vi "graph drivable paths.vi"(2 "updated max path lengths":u16[](array[numeric]), 3 "possible wheel angles":i8[](array[numeric])=[0, 0, 0, 0, 0, 0, 0, 0, 0, 0, 0, 0, 0, 0, 0, 0]) -> (0 "XY Graph":T1(graph))   [LabVIEW 2010]
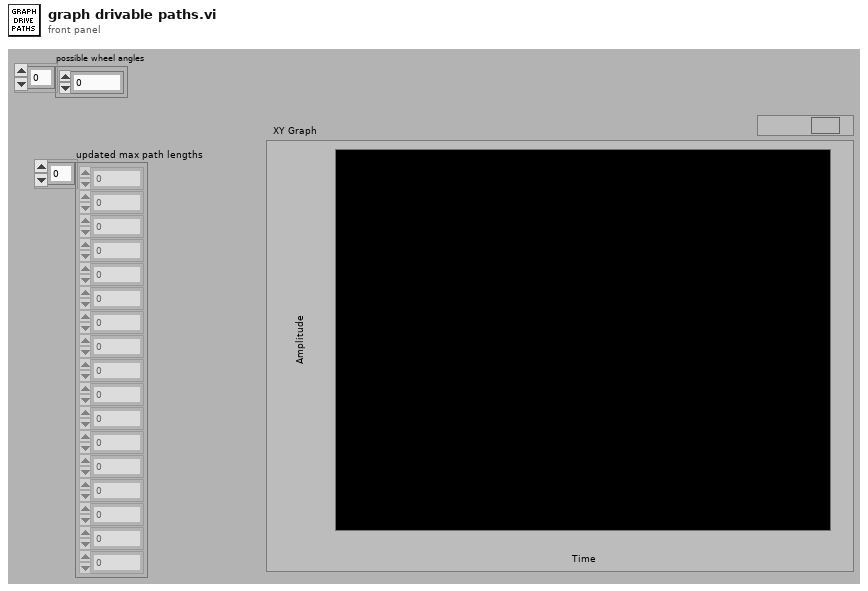
[diagram p1: front panel]
types:
  T1 = cluster{"New X Position":i16, "New Y Position":i16}[]
  T2 = cluster{"New X Position":i16, "New Y Position":i16}
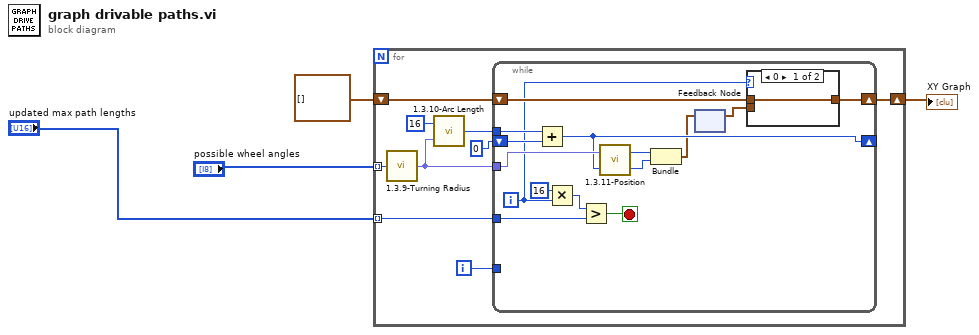
[diagram p0: block diagram]
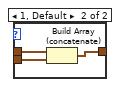
[diagram p2: hidden frame]
diagram:
  n1 = for {
    tunnel: "possible wheel angles" -> [w9] mode=indexing
    tunnel: "updated max path lengths" -> [w7] mode=indexing
    shift-right: [w6] -> w4
    shift-left: T1 [] -> [w5]
    i -> [w8]
    n2 = call "1.3.9-Turning Radius.vi"("Wheel Angle"=w9) -> ("Turning Radius (in)"=w13:fxp<+/-,22,12>)
    n3 = call "1.3.10-Arc Length.vi"("Turning Radius (in)"=w13, "Distance Along Arc"=u16 16) -> ("arc length angle"=w11:u16)
    n4 = while {
      tunnel: w13 -> [w27]
      tunnel: w11 -> [w28]
      shift-right: [w20] -> _
      shift-left: u16 0 ("arc length angle") -> [w26]
      tunnel: w8 -> [_]
      tunnel: w7 -> [w25]
      shift-right: [w21] -> w6
      shift-left: w5 -> [w22]
      i -> [w14]
      stop <- w19 stop-if-true
      n5 = Add(x=w28, y=w26) -> (x+y=w20:u16)
      n6 = Multiply(x=16, y=w14) -> (x*y=w18:i32)
      n7 = Greater?(x=w18, y=w25) -> (0:w19:bool)
      n8 = call "1.3.11-Position.vi"("arc length angle"=w20, "Turning Radius (in)"=w27) -> ("New Y Position"=w23:i16, "New X Position"=w24:i16)
      n9 = Bundle("New X Position"=w24, "New Y Position"=w23) -> (w16:T2)  [unwired: 1 in]
      n10 = feedback-in #1(w16) -> ()
      n11 = feedback #1() -> (w15:T2)  [unwired: 1 in]
      n12 = case shown="0" w14 {
        tunnel: w22 -> [w29 w32]
        tunnel: [w29 w31] -> w21
        tunnel: w15 -> [_ w30]
        frame 0 {
        }
        frame 1, Default {
          n13 = Build Array (concatenate)(w32, w30) -> (w31:T1)
        }
      }
    }
  }
  "XY Graph" <- w4
